vi "15- Addition of 2 input strings.vi"() -> ()   [LabVIEW 2019]
panel:
  out "Output string":string
  in  "Input string 2":string
  in  "Input string 1":string
  # "ADDITION OF 2 INPUT STRINGS"
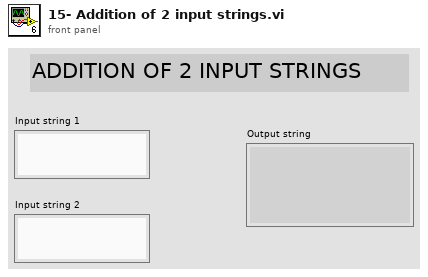
[diagram p1: front panel]
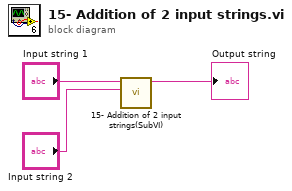
[diagram p0: block diagram]
diagram:
  n1 = call "15- Addition of 2 input strings(SubVI).vi"("Input string 2"="Input string 2", "Input string 1"="Input string 1") -> ("Output string"=→"Output string":string)  [unwired: 9 in]
